vi "createDirectoriesRemote.vi"(8 "error in (no error)":errorcluster, 10 "TimeStamp":string, 11 "FileNeologist in":refnum<class "FileNeologist.lvclass">) -> (0 "error out":errorcluster, 3 "FileNeologist out":refnum<class "FileNeologist.lvclass">)   [LabVIEW 2009, in "Tools.lvlib" / "Filing.lvlib" / "FileNeologist.lvclass"]
uses:
  FileNeologist.lvclass
  FileNeologist.lvclass/FileNeologist.ctl
  FileSystem/FileSystem.lvclass
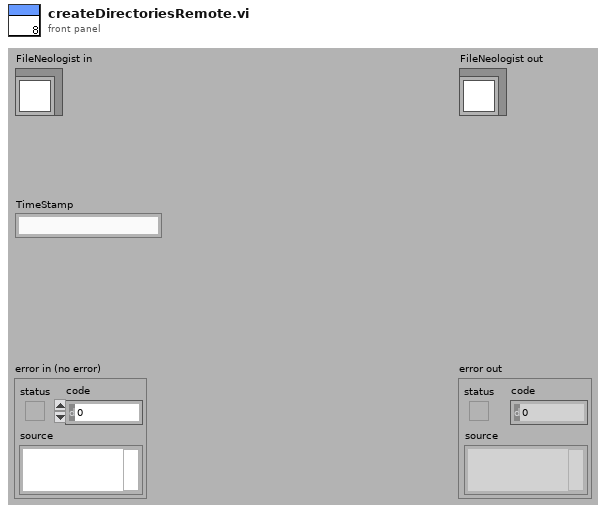
[diagram p1: front panel]
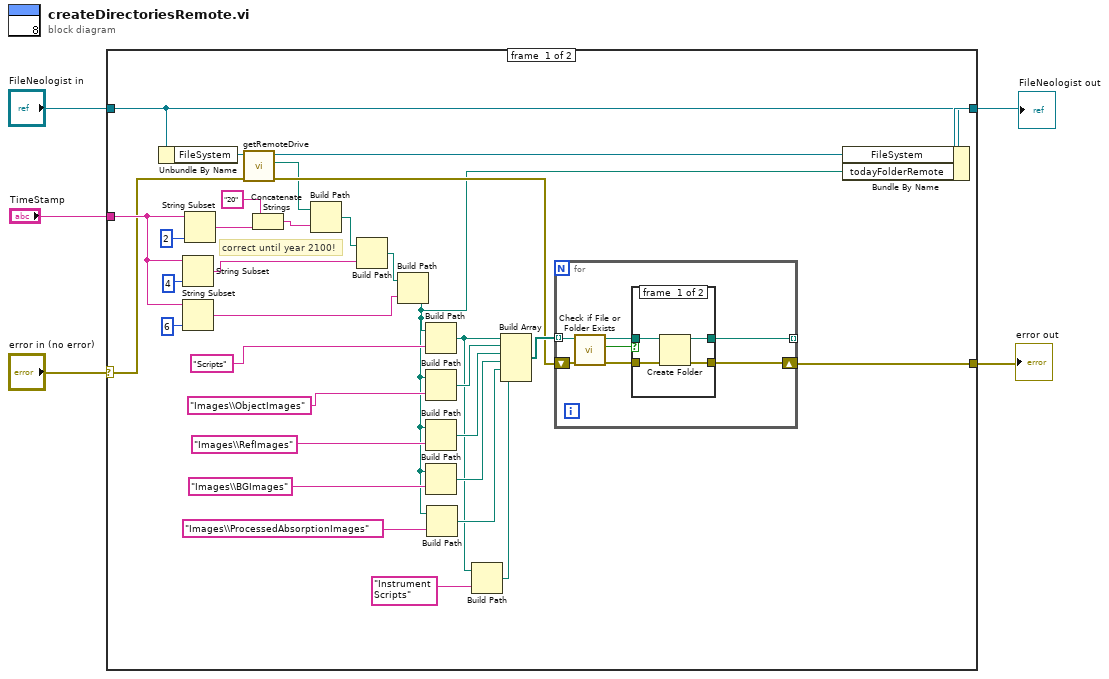
[diagram p0: block diagram]
diagram:
  n1 = case shown="No Error" "error in (no error)" {
    selector: "error in (no error)" -> [w10 w53]
    tunnel: [w23 w53] -> w4
    tunnel: [w22 w52] -> w2
    tunnel: "FileNeologist in" -> [w12 w52]
    tunnel: "TimeStamp" -> [w35 _]
    frame #0 {
      # "correct until year 2100!"
      n2 = Unbundle By Name(w12) -> ("FileSystem"=w11:refnum<class "FileSystem.lvclass">)
      n3 = String Subset(string=w35, length (rest)=4) -> (substring=w33:string)  [unwired: 1 in]
      n4 = String Subset(string=w35, length (rest)=6) -> (substring=w31:string)  [unwired: 1 in]
      n5 = String Subset(string=w35, length (rest)=2) -> (substring=w21:string)  [unwired: 1 in]
      n6 = call "getRemoteDrive.vi"("error in (no error)"=w10, "FileSystem in"=w11) -> ("error out"=w9:errorcluster, "RemoteDrive"=w8:path, "FileSystem out"=w7:refnum<class "FileSystem.lvclass">)  [unwired: 7 in]
      n7 = Concatenate Strings("20", w21) -> (w19:string)
      n8 = Build Path(base path=w8, name or relative path=w19) -> (appended path=w34:path)
      n9 = Build Path(base path=w34, name or relative path=w33) -> (appended path=w32:path)
      n10 = Build Path(base path=w32, name or relative path=w31) -> (appended path=w6:path)
      n11 = Build Path(base path=w6, name or relative path="Scripts") -> (appended path=w15:path)
      n12 = Build Path(base path=w6, name or relative path="Images\\ObjectImages") -> (appended path=w28:path)
      n13 = Build Path(base path=w6, name or relative path="Images\\RefImages") -> (appended path=w27:path)
      n14 = Build Path(base path=w6, name or relative path="Images\\BGImages") -> (appended path=w26:path)
      n15 = Build Path(base path=w6, name or relative path="Images\\ProcessedAbsorptionImages") -> (appended path=w25:path)
      n16 = Build Path(base path=w15, name or relative path="Instrument Scripts") -> (appended path=w13:path)
      n17 = Build Array(w15, w28, w27, w26, w25, w13) -> (w24:path[])
      n18 = for {
        tunnel: w24 -> [w42] mode=indexing
        shift-right: [w40] -> w23
        shift-left: w9 -> [w41]
        tunnel: [w39] -> _ mode=indexing
        n19 = call <vilib>:"Check if File or Folder Exists.vi"("error in (no error)"=w41, "path"=w42) -> ("error out"=w43:errorcluster, "file or folder exists?"=w45:bool, "dup path"=w44:path)  [unwired: 7 in]
        n20 = case shown="False" w45 {
          tunnel: w44 -> [w49 w51]
          tunnel: [w46 w51] -> w39
          tunnel: w43 -> [w48 w50]
          tunnel: [w47 w50] -> w40
          frame #0 {
            n21 = Create Folder(path (use dialog)=w49, error in=w48) -> (created path=w46:path, error out=w47:errorcluster)  [unwired: 1 in, 1 out]
          }
          frame #1 {
          }
        }
      }
      n22 = Bundle By Name(cluster=w12, "FileSystem"=w7, "todayFolderRemote"=w6) -> (w22:refnum<class "FileNeologist.lvclass">)
    }
    frame #1 {
    }
  }
  "error out" <- w4
  "FileNeologist out" <- w2
